vi "Write-To-Bin.vi"(0 "Weights Cluster":T1) -> ()   [LabVIEW 2020]
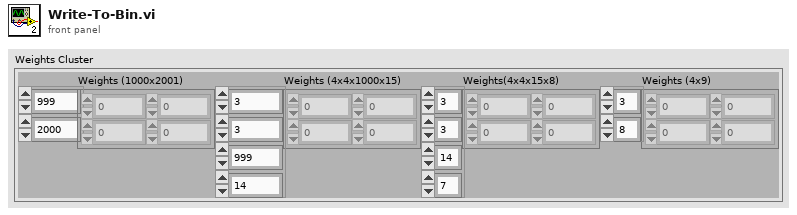
[diagram p1: front panel]
types:
  T1 = cluster{"Weights (1000x2001)":dbl[][], "Weights (4x4x1000x15)":dbl[][][][], "Weights(4x4x15x8)":dbl[][][][], "Weights (4x9)":dbl[][]}
  T2 = enum16{"open", "replace", "create", "open or create", "replace or create", "replace or create with confirmation"}
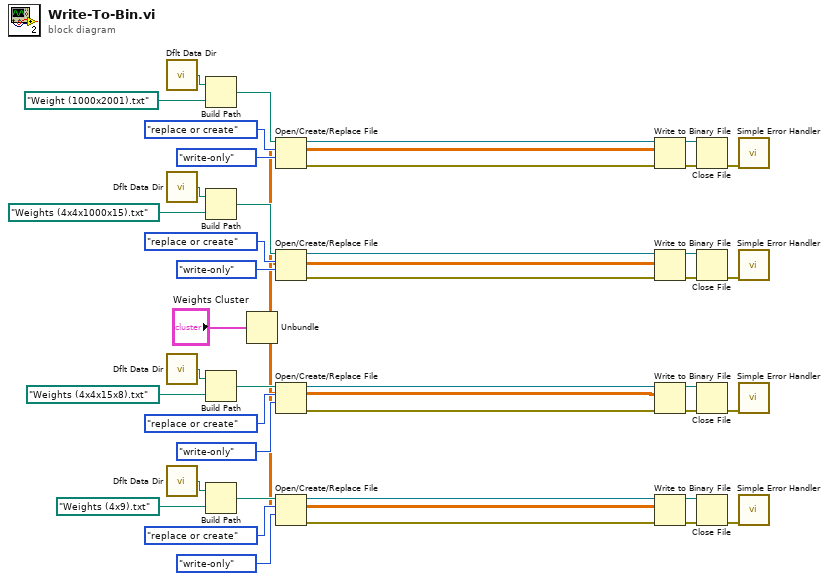
[diagram p0: block diagram]
diagram:
  n1 = call <vilib>:"Dflt Data Dir.vi"() -> ("App:Default Data Directory"=w41:path)
  n2 = call <vilib>:"Dflt Data Dir.vi"() -> ("App:Default Data Directory"=w31:path)
  n3 = call <vilib>:"Dflt Data Dir.vi"() -> ("App:Default Data Directory"=w21:path)
  n4 = call <vilib>:"Dflt Data Dir.vi"() -> ("App:Default Data Directory"=w11:path)
  n5 = Build Path(base path=w41, name or relative path=path "Weight (1000x2001).txt" ("default name")) -> (appended path=w35:path)
  n6 = Build Path(base path=w31, name or relative path=path "Weights (4x4x1000x15).txt" ("default name")) -> (appended path=w25:path)
  n7 = Build Path(base path=w21, name or relative path=path "Weights (4x4x15x8).txt" ("default name")) -> (appended path=w15:path)
  n8 = Build Path(base path=w11, name or relative path=path "Weights (4x9).txt" ("default name")) -> (appended path=w5:path)
  n9 = Unbundle("Weights Cluster") -> ("Weights (1000x2001)"=w4:dbl[][], "Weights (4x4x1000x15)"=w3:dbl[][][][], "Weights(4x4x15x8)"=w2:dbl[][][][], "Weights (4x9)"=w1:dbl[][])
  n10 = Open/Create/Replace File(file path (use dialog)=w35, operation (0:open)=T2."replace or create", access (0:read/write)=enum16{"read/write", "read-only", "write-only"}."write-only") -> (refnum out=w40:refnum<file>, error out=w39:errorcluster)  [unwired: 1 in, 3 out]
  n11 = Open/Create/Replace File(file path (use dialog)=w25, operation (0:open)=T2."replace or create", access (0:read/write)=enum16{"read/write", "read-only", "write-only"}."write-only") -> (refnum out=w30:refnum<file>, error out=w29:errorcluster)  [unwired: 1 in, 3 out]
  n12 = Open/Create/Replace File(file path (use dialog)=w15, operation (0:open)=T2."replace or create", access (0:read/write)=enum16{"read/write", "read-only", "write-only"}."write-only") -> (refnum out=w20:refnum<file>, error out=w19:errorcluster)  [unwired: 1 in, 3 out]
  n13 = Open/Create/Replace File(file path (use dialog)=w5, operation (0:open)=T2."replace or create", access (0:read/write)=enum16{"read/write", "read-only", "write-only"}."write-only") -> (refnum out=w10:refnum<file>, error out=w9:errorcluster)  [unwired: 1 in, 3 out]
  n14 = Write to Binary File(file (use dialog)=w40, data=w4, error in=w39) -> (refnum out=w37:refnum<file>, error out=w38:errorcluster)  [unwired: 3 in, 1 out]
  n15 = Write to Binary File(file (use dialog)=w30, data=w3, error in=w29) -> (refnum out=w27:refnum<file>, error out=w28:errorcluster)  [unwired: 3 in, 1 out]
  n16 = Write to Binary File(file (use dialog)=w20, data=w2, error in=w19) -> (refnum out=w17:refnum<file>, error out=w18:errorcluster)  [unwired: 3 in, 1 out]
  n17 = Write to Binary File(file (use dialog)=w10, data=w1, error in=w9) -> (refnum out=w7:refnum<file>, error out=w8:errorcluster)  [unwired: 3 in, 1 out]
  n18 = Close File(refnum=w37, error in=w38) -> (error out=w36:errorcluster)  [unwired: 1 out]
  n19 = Close File(refnum=w27, error in=w28) -> (error out=w26:errorcluster)  [unwired: 1 out]
  n20 = Close File(refnum=w17, error in=w18) -> (error out=w16:errorcluster)  [unwired: 1 out]
  n21 = Close File(refnum=w7, error in=w8) -> (error out=w6:errorcluster)  [unwired: 1 out]
  n22 = call <vilib>:"Simple Error Handler.vi"("error in (no error)"=w36) -> ()  [unwired: 1 in, 8 out]
  n23 = call <vilib>:"Simple Error Handler.vi"("error in (no error)"=w26) -> ()  [unwired: 1 in, 8 out]
  n24 = call <vilib>:"Simple Error Handler.vi"("error in (no error)"=w16) -> ()  [unwired: 1 in, 8 out]
  n25 = call <vilib>:"Simple Error Handler.vi"("error in (no error)"=w6) -> ()  [unwired: 1 in, 8 out]
